vi "Write_JSON.vi"(6 "error in":errorcluster caption="entrée d'erreur") -> (0 "error out":errorcluster caption="sortie d'erreur")   [LabVIEW 2026]
uses:
  FGV/TypeDef_FGV.ctl
  <vilib>/addons/_JKI.lib/Serialization/JSON/JKI JSON Serialization.lvlib
panel:
  out "JSON String":string
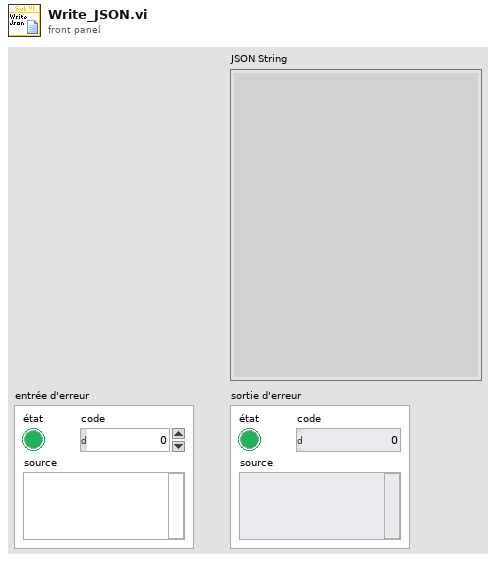
[diagram p1: front panel]
types:
  T1 = typedef "TypeDef_FGV.ctl" = enum16{"Initialize", "Write", "Read", "Read_File", "Write_to_File"}
  T2 = typedef "TypeDef_Array_ChannelCluster.ctl" = cluster{"Laser":enum16{"405 nm", "455 nm", "488 nm", "561 nm", "640 nm"}, "Power (%)":u8, "Exposure time (s)":dbl, "Channel ON-OFF":bool, "Polar ON-OFF":bool, "Filter":u16}[]
  T3 = cluster{"Sample rate OUT":u32, "Start/Live (0/1) OUT":bool, "Channel_Cluster_Array OUT":T2, "Readout time (s) OUT":dbl, "Extra time for FW (s) OUT":dbl, "Polar_Array OUT":dbl[][], "Z_Array OUT":dbl[], "Multipositions current OUT":dbl[], "Multipositions array OUT":dbl[][]}
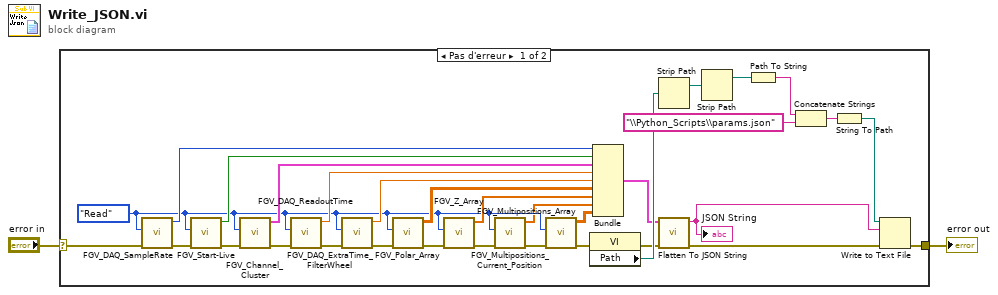
[diagram p0: block diagram]
diagram:
  n1 = case shown="Pas d'erreur" "error in" {
    selector: "error in" -> [w34 w35]
    tunnel: [w17 w35] -> w1
    frame No Error {
      w6 = TypeDef_FGV."Read" ("Action")
      n2 = call "FGV_DAQ_SampleRate.vi"("error in"=w34, "Action"=w6) -> ("error out"=w33:errorcluster, "Sample rate OUT"=w16:u32)  [unwired: 8 in]
      n3 = call "FGV_Start-Live.vi"("error in"=w33, "Action"=w6) -> ("error out"=w32:errorcluster, "Start/Live (0/1) OUT"=w15:bool)  [unwired: 8 in]
      n4 = call "FGV_Channel_Cluster.vi"("error in"=w32, "Action"=w6) -> ("error out"=w31:errorcluster, "Channel_Cluster_Array OUT"=w14:T2)  [unwired: 8 in]
      n5 = call "FGV_DAQ_ReadoutTime.vi"("error in"=w31, "Action"=w6) -> ("error out"=w30:errorcluster, "Readout time (s) OUT"=w13:dbl)  [unwired: 8 in]
      n6 = call "FGV_DAQ_ExtraTime_FilterWheel.vi"("error in"=w30, "Action"=w6) -> ("error out"=w29:errorcluster, "Extra time for FW (s) OUT"=w12:dbl)  [unwired: 8 in]
      n7 = call "FGV_Polar_Array.vi"("error in"=w29, "Action"=w6) -> ("error out"=w28:errorcluster, "Polar_Array OUT"=w11:dbl[][])  [unwired: 7 in, 1 out]
      n8 = call "FGV_Z_Array.vi"("error in"=w28, "Action"=w6) -> ("error out"=w7:errorcluster, "Z_Array OUT"=w10:dbl[])  [unwired: 7 in, 1 out]
      n9 = call "FGV_Multipositions_Current_Position.vi"("error in"=w7, "Action"=w6) -> ("error out"=w5:errorcluster, "Multipositions current OUT"=w4:dbl[])  [unwired: 8 in]
      n10 = call "FGV_Multipositions_Array.vi"("error in"=w5, "Action"=w6) -> ("error out"=w18:errorcluster, "Multipositions array OUT"=w3:dbl[][])  [unwired: 7 in, 1 out]
      n11 = property class="VI"(error in=w18) -> (error out=w21:errorcluster, "Path"=w27:path)  [unwired: 1 in, 1 out]
      n12 = Bundle("Sample rate OUT"=w16, "Start/Live (0/1) OUT"=w15, "Channel_Cluster_Array OUT"=w14, "Readout time (s) OUT"=w13, "Extra time for FW (s) OUT"=w12, "Polar_Array OUT"=w11, "Z_Array OUT"=w10, "Multipositions current OUT"=w4, "Multipositions array OUT"=w3) -> (w22:T3)  [unwired: 1 in]
      n13 = Strip Path(path=w27) -> (stripped path=w8:path)  [unwired: 1 out]
      n14 = call <vilib>:"Flatten To JSON String.vi"("error in"=w21, "Variant"=w22) -> ("error out"=w19:errorcluster, "JSON String"=w20:string)  [unwired: 8 in]
      "JSON String" <- w20
      n15 = Strip Path(path=w8) -> (stripped path=w9:path)  [unwired: 1 out]
      n16 = Path To String(path=w9) -> (string=w25:string)
      n17 = Concatenate Strings(w25, "\\Python_Scripts\\params.json" ("string")) -> (w24:string)
      n18 = String To Path(string=w24) -> (path=w23:path)
      n19 = Write to Text File(file (use dialog)=w23, text=w20, error in=w19) -> (error out=w17:errorcluster)  [unwired: 1 in, 2 out]
    }
    frame Error {
    }
  }
  "error out" <- w1
